vi "MotorPWM_B(SubVI).vi"(10 "Stop Vi":bool, 11 "Duty Cycle (-100 to + 100)":dbl) -> ()   [LabVIEW 2017]
uses:
  <vilib>/myRIO/Common/Instrument Driver Framework/myRIO v1.0/DIO/typedefs/DIO Channels Enum.ctl
  <vilib>/myRIO/Common/Instrument Driver Framework/myRIO v1.0/DIO/typedefs/DIO Channels List.ctl
  <vilib>/myRIO/Common/Instrument Driver Framework/Utilities/typedefs/Generic FPGA Reference.ctl
  <vilib>/myRIO/Common/Instrument Driver Framework/Utilities/typedefs/myRIO v1.0 Reference.ctl
  <vilib>/myRIO/Common/Instrument Driver Framework/Utilities/typedefs/Hardware Version Enum.ctl
  <vilib>/myRIO/Common/Instrument Driver Framework/Utilities/typedefs/myRIO Generic Hardware Reference.ctl
  <vilib>/myRIO/Instrument Drivers/Onboard IO/DIO/typedefs/DIO Reference.ctl
  <vilib>/myRIO/Instrument Drivers/Onboard IO/DIO/DIO.lvlib
  <vilib>/myRIO/Instrument Drivers/Onboard IO/DIO/vis/Write.vi
  <vilib>/userdefined/High Color/nirio_resource_hc.ctl
  <vilib>/myRIO/Common/Instrument Driver Framework/myRIO v1.0/DIO/vis/myRIO v1.1 Open DIO.vi
  <vilib>/myRIO/Instrument Drivers/Onboard IO/DIO/vis/myRIO DIO Open.xnode
  <vilib>/myRIO/Common/Instrument Driver Framework/Utilities/vis/Is FPGA Ref Available.vi
  <vilib>/myRIO/Express VI/Onboard IO/DO/DO Express VI.xnode
  <vilib>/myRIO/Express VI/Onboard IO/PWM/PWM Express VI.xnode
  <vilib>/myRIO/Instrument Drivers/Onboard IO/PWM/vis/Set Duty Cycle and Frequency.vi
  <vilib>/myRIO/Instrument Drivers/Onboard IO/PWM/PWM.lvlib
  <vilib>/myRIO/Instrument Drivers/Onboard IO/PWM/typedefs/PWM Configuration.ctl
  <vilib>/myRIO/Common/Instrument Driver Framework/myRIO v1.0/PWM/typedefs/PWM Channels Enum.ctl
  <vilib>/myRIO/Instrument Drivers/Onboard IO/PWM/typedefs/PWM Reference.ctl
  <vilib>/myRIO/Instrument Drivers/Onboard IO/PWM/vis/myRIO PWM Open.xnode
  <vilib>/myRIO/Common/Instrument Driver Framework/myRIO v1.0/PWM/vis/myRIO v1.1 Open PWM.vi
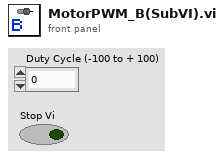
[diagram p1: front panel]
types:
  T1 = typedef "DIO.lvlib/DIO Reference.ctl" = cluster{"myRIO Reference":T2, "DIO Channels List":T6}
  T2 = typedef "myRIO Generic Hardware Reference.ctl" = cluster{"myRIO Model":T3, "myRIO Hardware Reference":T4}
  T3 = typedef "Hardware Version Enum.ctl" = enum16{"Unknown", "myRIO-1900", "myRIO-1950", "roboRIO", "NI ELVIS RIO CM"}
  T4 = typedef "myRIO v1.0 Reference.ctl" = cluster{"Generic FPGA Reference":T5, "Allow multiple opens":bool}
  T5 = typedef "Generic FPGA Reference.ctl" = refnum<k20>
  T6 = typedef "DIO Channels List.ctl" = T7[]
  T7 = typedef "DIO Channels Enum.ctl" = enum16{"Not Connected", "C/DIO0", "C/DIO1", "C/DIO2", "C/DIO3", "C/DIO4", "C/DIO5", "C/DIO6", "C/DIO7", "A/DIO0", "A/DIO1", "A/DIO2", "A/DIO3", "A/DIO4", "A/DIO5", "A/DIO6", "A/DIO7", "A/DIO8", "A/DIO9", "A/DIO10", "A/DIO11", "A/DIO12", "A/DIO13", "A/DIO14", "A/DIO15", "B/DIO0", "B/DIO1", "B/DIO2", "B/DIO3", "B/DIO4", "B/DIO5", "B/DIO6", "B/DIO7", "B/DIO8", "B/DIO9", "B/DIO10", "B/DIO11", "B/DIO12", "B/DIO13", "B/DIO14", "B/DIO15", "LED0", "LED1", "LED2", "LED3", "Button0", "DIO/DIO0", "DIO/DIO1", "DIO/DIO2", "DIO/DIO3", "DIO/DIO4", "DIO/DIO5", "DIO/DIO6", "DIO/DIO7", "DIO/DIO8", "DIO/DIO9", "SPI/CS0", "SPI/CS1", "SPI/CS2", "SPI/CS3", "LED RADIO (Green)", "LED RADIO (Red)", "LED COMM (Green)", "LED COMM (Red)", "LED MODE (Green)", "LED MODE (Red)"}
  T8 = typedef "nirio_resource_hc.ctl" = tag
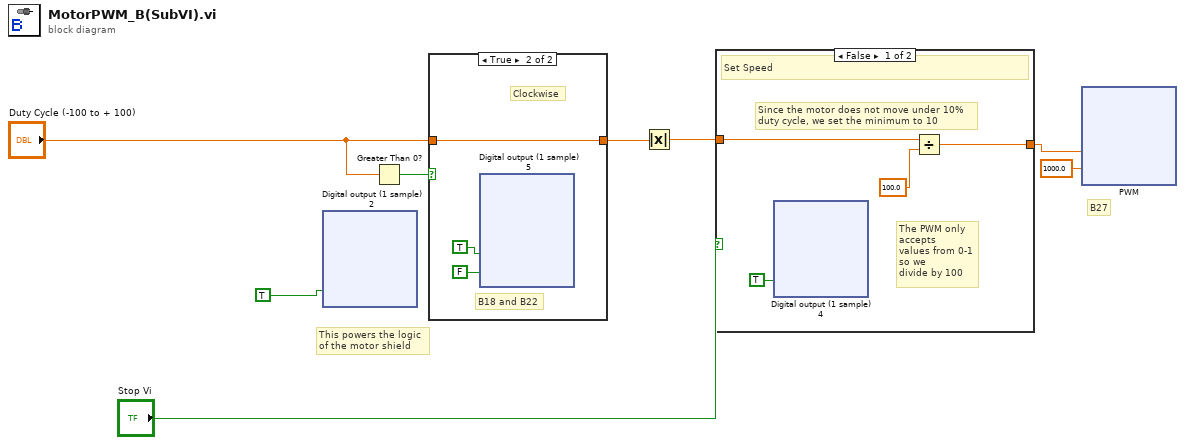
[diagram p0: block diagram]
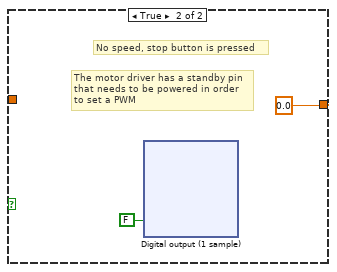
[diagram p2: hidden frame]
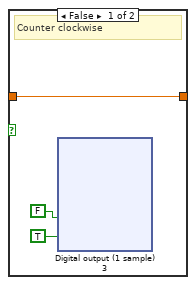
[diagram p3: hidden frame]
diagram:
  # "B27"
  # "This powers the logic\nof the motor shield"
  n1 = xnode "Digital output (1 sample) 2"("Driver Vcc (A/DIO3 (Pin 17))"=TRUE) -> ()  [unwired: 1 in, 1 out]
  n2 = Greater Than 0?(x="Duty Cycle (-100 to + 100)") -> (x > 0?=w7:bool)
  n3 = case shown="True" w7 {
    tunnel: "Duty Cycle (-100 to + 100)" -> [w11 w50]
    tunnel: [w11 w50] -> w6
    frame False {
      # "Counter clockwise"
      n4 = xnode "Digital output (1 sample) 3"("BIN2 (B/DIO11 (Pin 18))"=FALSE ("STBY (A/DIO2 (Pin 15))"), "BIN1 (B/DIO12 (Pin 22))"=TRUE ("STBY (A/DIO2 (Pin 15))")) -> ()  [unwired: 1 in, 1 out]
    }
    frame True {
      # "B18 and B22"
      # "Clockwise"
      n5 = xnode "Digital output (1 sample) 5"("BIN2 (B/DIO11 (Pin 18))"=TRUE ("STBY (A/DIO2 (Pin 15))"), "BIN1 (B/DIO12 (Pin 22))"=FALSE ("STBY (A/DIO2 (Pin 15))")) -> ()  [unwired: 1 in, 1 out]
    }
  }
  n6 = Absolute Value(x=w6) -> (abs(x)=w5:dbl)
  n7 = case shown="False" "Stop Vi" {
    tunnel: w5 -> [w88 _]
    tunnel: [w87 0.0] -> w2
    frame False {
      # "Since the motor does not move under 10%\nduty cycle, we set the minimum to 10"
      # "The PWM only\naccepts\nvalues from 0-1\nso we\ndivide by 100"
      # "Set Speed"
      n8 = xnode "Digital output (1 sample) 4"("STBY (A/DIO2 (Pin 15))"=TRUE) -> ()  [unwired: 1 in, 1 out]
      n9 = Divide(x=w88, y=100.0) -> (x/y=w87:dbl)
    }
    frame True {
      # "No speed, stop button is pressed"
      # "The motor driver has a standby pin\nthat needs to be powered in order\nto set a PWM"
      n10 = xnode "Digital output (1 sample)"("STBY (A/DIO2 (Pin 15))"=FALSE) -> ()  [unwired: 1 in, 1 out]
    }
  }
  n11 = xnode "PWM"("Duty Cycle"=w2, "Frequency [Hz]"=1000.0) -> ()  [unwired: 1 in, 1 out]
